vi "Attitude Indicator Facade.vi"(0 "Data In":T6, 2 "Display State In":T2={"Draw Options"={"Text Color"=16777238, "Wing Color"=16751616, "Dial Outline Color"=13816530, "Sky Color"=3381759, "Ground Color"=8213043, "Horizon Line Color"=16777225, "Outline Color"=0, "Dial Background Color"=5987163, "Draw Wings"=TRUE, "Draw Text"=TRUE, "Font Name"="Helvetica", "Angle units"=enum."Radians"}}, 3 "Container State":T5) -> (6 "Data Out":T6, 7 "Display State Out":T2={"Draw Options"={"Text Color"=16777238, "Wing Color"=16751616, "Dial Outline Color"=13816530, "Sky Color"=3381759, "Ground Color"=8213043, "Horizon Line Color"=16777225, "Outline Color"=0, "Dial Background Color"=5987163, "Draw Wings"=TRUE, "Draw Text"=TRUE, "Font Name"="Helvetica", "Angle units"=enum."Radians"}}, 8 "Action":T1)   [LabVIEW 2017, in "Attitude Indicator.xctl"]
uses:
  <vilib>/robotics/Controls/Attitude Indicator/Attitude Indicator.xctl
  <vilib>/robotics/Controls/Attitude Indicator/_Attitude Indicator Support Files/Attitude Indicator Data.ctl
  <vilib>/_xctls/Container State.ctl
  <vilib>/robotics/Controls/Attitude Indicator/_Attitude Indicator Support Files/Attitude Indicator State.ctl
  <vilib>/robotics/Controls/Attitude Indicator/Attitude Picture/Draw Options.ctl
  <vilib>/robotics/Controls/Utilities/Angle Units.ctl
  <vilib>/_xctls/Action.ctl
  <vilib>/_xctls/XControlSupport.lvlib
  <vilib>/robotics/Controls/Utilities/NI_Robotics_Control Utilities.lvlib
  <vilib>/robotics/Controls/Attitude Indicator/Attitude Picture/NI_Robotics_Attitude Picture.lvlib
panel:
  out "2D Picture":picture
types:
  T1 = typedef "XControlSupport.lvlib/Action.ctl" = cluster{"Data Changed?":bool, "State Changed?":bool, "Action Name":string}
  T2 = typedef "Attitude Indicator.xctl/Attitude Indicator State.ctl" = cluster{"Draw Options":T3}
  T3 = typedef "NI_Robotics_Attitude Picture.lvlib/Draw Options.ctl" = cluster{"Text Color":u32, "Wing Color":u32, "Dial Outline Color":u32, "Sky Color":u32, "Ground Color":u32, "Horizon Line Color":u32, "Outline Color":u32, "Dial Background Color":u32, "Draw Wings":bool, "Draw Text":bool, "Font Name":string, "Angle units":T4}
  T4 = typedef "NI_Robotics_Control Utilities.lvlib/Angle Units.ctl" = enum16{"Radians", "Degrees"}
  T5 = typedef "XControlSupport.lvlib/Container State.ctl" = cluster{"Indicator?":bool, "Run Mode?":bool, " Refnum":refnum<vi>}
  T6 = typedef "Attitude Indicator.xctl/Attitude Indicator Data.ctl" = cluster{"Roll":dbl, "Pitch":dbl}
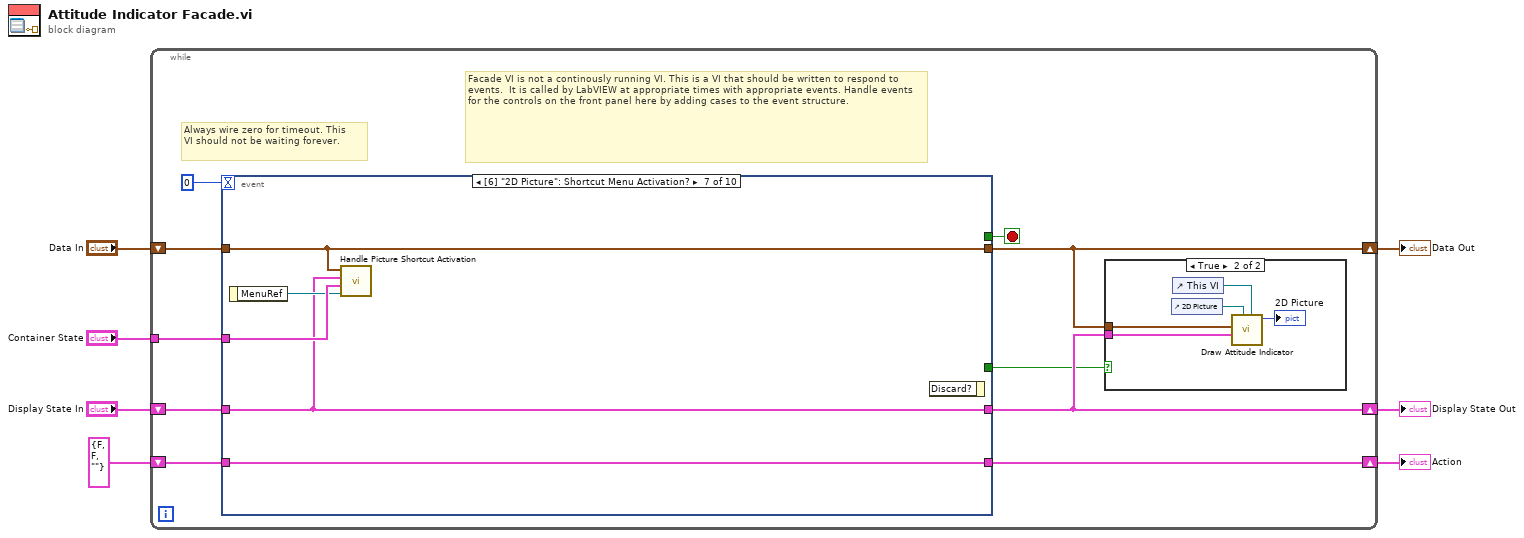
[diagram p0: block diagram]
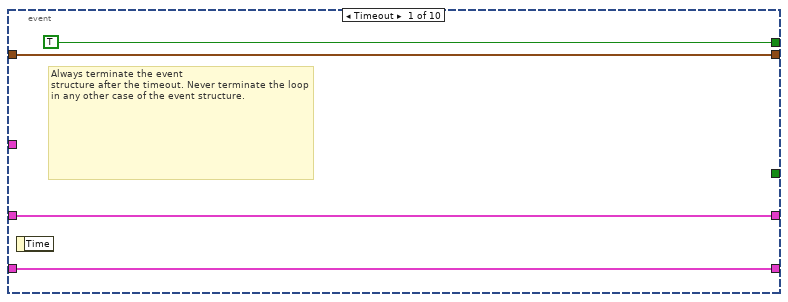
[diagram p3: hidden frame]
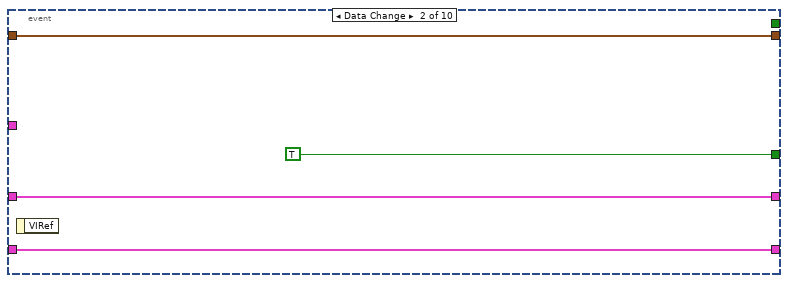
[diagram p4: hidden frame]
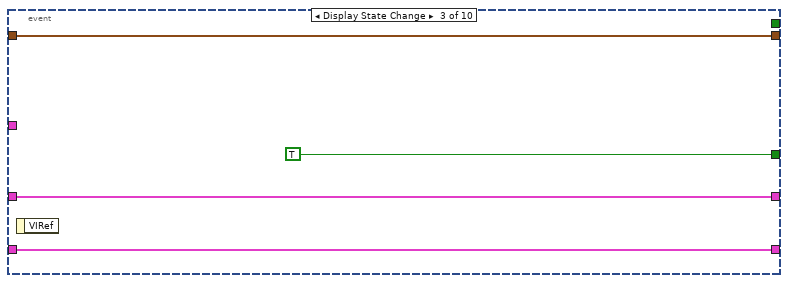
[diagram p5: hidden frame]
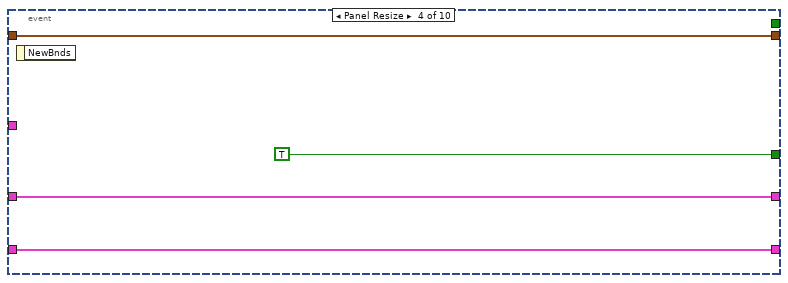
[diagram p6: hidden frame]
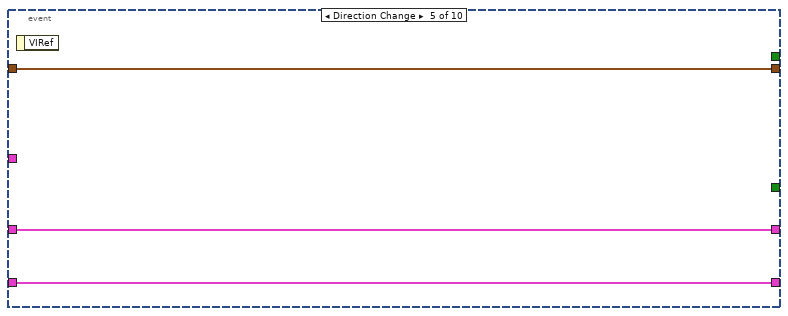
[diagram p7: hidden frame]
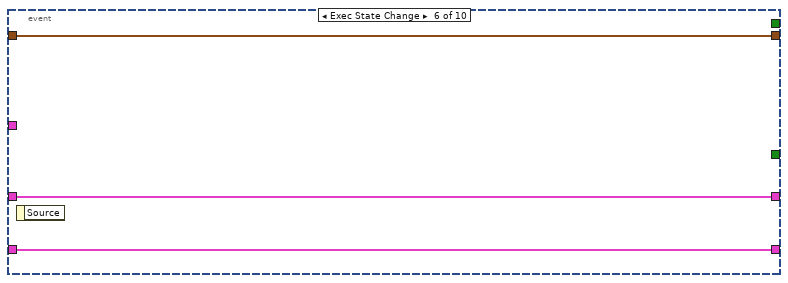
[diagram p8: hidden frame]
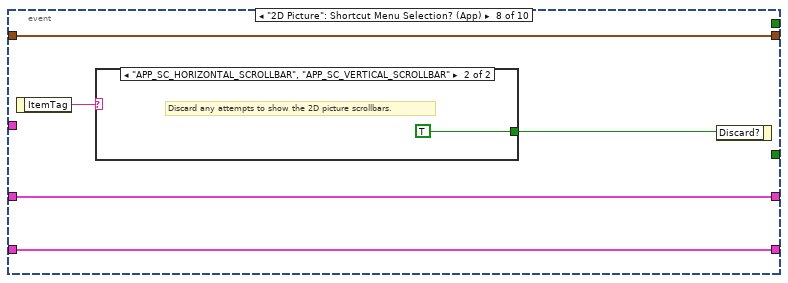
[diagram p9: hidden frame]
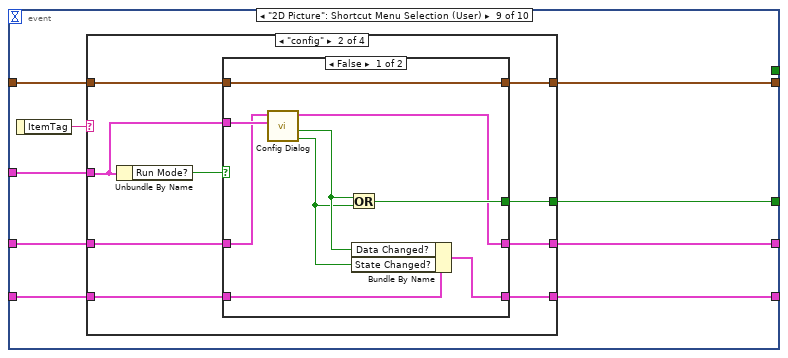
[diagram p11: hidden frame]
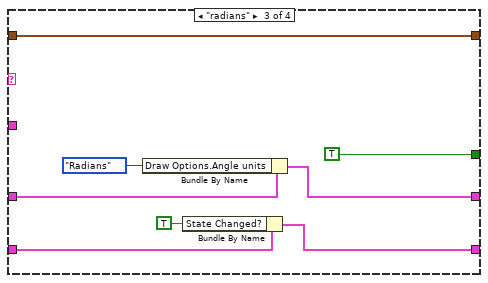
[diagram p14: hidden frame]
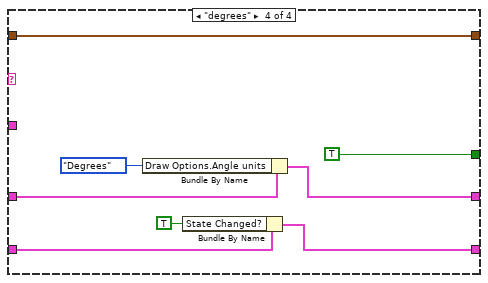
[diagram p15: hidden frame]
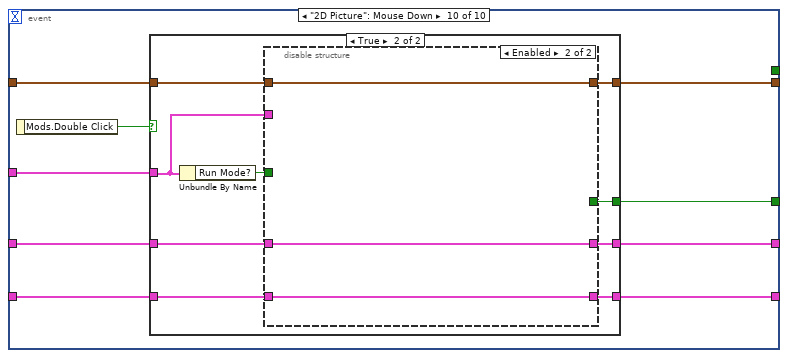
[diagram p16: hidden frame]
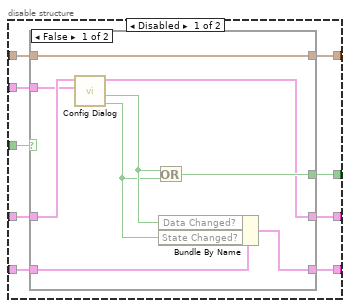
[diagram p18: hidden frame]
diagram:
  n1 = while {
    shift-right: [w10] -> w4
    shift-left: "Display State In" -> [w17]
    tunnel: "Container State" -> [w14]
    shift-right: [w11] -> w7
    shift-left: "Data In" -> [w13]
    shift-right: [w9] -> w1
    shift-left: T1 {"Data Changed?"=FALSE, "State Changed?"=FALSE, "Action Name"=""} ("Action") -> [w12]
    stop <- w16 stop-if-true
    # "Facade VI is not a continously running VI. This is a VI that should be written to respond to events.  It is called by LabVIEW at appropriate times with appropriate events. Handle events for the controls on the front panel here by adding cases to the event structure."
    # "Always wire zero for timeout. This\nVI should not be waiting forever."
    n2 = event shown="[6] \"2D Picture\": Shortcut Menu Activation?" {
      selector: _ -> [_ _ _ _ _ _ _ _ _ _]
      dyn-events: _ -> [_ _ _ _ _ _ _ _ _ _]
      timeout: 0 -> [_ _ _ _ _ _ _ _ _ _]
      tunnel: w17 -> [w25 w28 w32 w37 w41 w44 w45 w54 w61 w110]
      tunnel: [w25 w28 w32 w37 w41 w44 w45 w54 w60 w109] -> w10
      tunnel: [TRUE _ _ _ _ _ _ _ _ _] -> w16
      tunnel: w14 -> [_ _ _ _ _ _ w48 _ w56 w105]
      tunnel: w13 -> [w24 w29 w33 w38 w40 w43 w46 w53 w63 w112]
      tunnel: [w24 w29 w33 w38 w40 w43 w46 w53 w62 w111] -> w11
      tunnel: w12 -> [w23 w27 w31 w36 w39 w42 w49 w52 w59 w108]
      tunnel: [w23 w27 w31 w36 w39 w42 w49 w52 w58 w107] -> w9
      tunnel: [_ TRUE TRUE TRUE _ _ _ _ w57 w106] -> w8
      event Timeout {
        # "Always terminate the event\nstructure after the timeout. Never terminate the loop in any other case of the event structure."
        n3 = event-data() -> ()  [unwired: 1 in, 1 out]
      }
      event Data Change {
        n4 = event-data() -> ()  [unwired: 1 in, 1 out]
      }
      event Display State Change {
        n5 = event-data() -> ()  [unwired: 1 in, 1 out]
      }
      event Panel Resize {
        n6 = event-data() -> ()  [unwired: 1 in, 1 out]
      }
      event Direction Change {
        n7 = event-data() -> ()  [unwired: 1 in, 1 out]
      }
      event Exec State Change {
        n8 = event-data() -> ()  [unwired: 1 in, 1 out]
      }
      event "2D Picture": Shortcut Menu Activation? {
        n9 = event-data() -> ("MenuRef"=w47:refnum<k9>)  [unwired: 1 in]
        n10 = call <vilib>:"Handle Picture Shortcut Activation.vi"("MenuRef"=w47, "Container State"=w48, "state in"=w45, "data in"=w46) -> ()  [unwired: 8 in]
        n11 = event-data() -> ()  [unwired: 2 in, 1 out]
      }
      event "2D Picture": Shortcut Menu Selection? (App) {
        n12 = event-data() -> ("ItemTag"=w50:string)  [unwired: 1 in]
        n13 = case shown="\"APP_SC_HORIZONTAL_SCROLLBAR\", \"APP_SC_VERTICAL_SCROLLBAR\"" w50 {
          tunnel: [_ TRUE] -> w51
          frame Default {
          }
          frame "APP_SC_HORIZONTAL_SCROLLBAR", "APP_SC_VERTICAL_SCROLLBAR" {
            # "Discard any attempts to show the 2D picture scrollbars."
          }
        }
        n14 = event-data("Discard?"=w51) -> ()  [unwired: 1 in, 1 out]
      }
      event "2D Picture": Shortcut Menu Selection (User) {
        n15 = event-data() -> ("ItemTag"=w64:string)  [unwired: 1 in]
        n16 = case shown="\"config\"" w64 {
          tunnel: w63 -> [w67 w76 w96 w104]
          tunnel: [w67 w75 w96 w104] -> w62
          tunnel: w61 -> [w66 w74 w95 w103]
          tunnel: [w66 w73 w94 w102] -> w60
          tunnel: w59 -> [w65 w72 w92 w100]
          tunnel: [w65 w71 w91 w99] -> w58
          tunnel: [_ w70 TRUE TRUE] -> w57
          tunnel: w56 -> [_ w68 _ _]
          frame Default {
          }
          frame "config" {
            n17 = Unbundle By Name(w68) -> ("Run Mode?"=w69:bool)
            n18 = case shown="False" w69 {
              tunnel: w76 -> [w77 w88]
              tunnel: [w77 w88] -> w75
              tunnel: w74 -> [w78 w87]
              tunnel: [w80 w87] -> w73
              tunnel: w72 -> [w85 w86]
              tunnel: [w84 w86] -> w71
              tunnel: [w81 _] -> w70
              tunnel: w68 -> [w79 _]
              frame False {
                n19 = call <vilib>:"Config Dialog.vi"("Container State"=w79, "state in"=w78) -> ("state changed?"=w82:bool, "data changed?"=w83:bool, "state out"=w80:T2)  [unwired: 7 in]
                n20 = Or(x=w83, y=w82) -> (x .or. y?=w81:bool)
                n21 = Bundle By Name(cluster=w85, "Data Changed?"=w83, "State Changed?"=w82) -> (w84:T1)
              }
              frame True {
                # "Do not launch config dialog if xctl is in a running VI."
              }
            }
          }
          frame "radians" {
            n22 = Bundle By Name(cluster=w95, "Draw Options.Angle units"=Angle_Units."Radians") -> (w94:T2)
            n23 = Bundle By Name(cluster=w92, "State Changed?"=TRUE) -> (w91:T1)
          }
          frame "degrees" {
            n24 = Bundle By Name(cluster=w103, "Draw Options.Angle units"=Angle_Units."Degrees") -> (w102:T2)
            n25 = Bundle By Name(cluster=w100, "State Changed?"=TRUE) -> (w99:T1)
          }
        }
      }
      event "2D Picture": Mouse Down {
        n26 = event-data() -> ("Mods.Double Click"=w113:bool)  [unwired: 1 in]
        n27 = case shown="True" w113 {
          tunnel: w112 -> [w116 w125]
          tunnel: [w116 w124] -> w111
          tunnel: w110 -> [w115 w123]
          tunnel: [w115 w122] -> w109
          tunnel: w108 -> [w114 w121]
          tunnel: [w114 w120] -> w107
          tunnel: [_ w119] -> w106
          tunnel: w105 -> [_ w117]
          frame False {
          }
          frame True {
            n28 = Unbundle By Name(w117) -> ("Run Mode?"=w118:bool)
            n29 = disable-structure shown="Enabled" {
              disable-tunnel: w125 -> [w134 w149]
              disable-tunnel: [w133 w149] -> w124
              disable-tunnel: w123 -> [w132 w148]
              disable-tunnel: [w131 w148] -> w122
              disable-tunnel: w121 -> [w130 w147]
              disable-tunnel: [w129 w147] -> w120
              disable-tunnel: [w128 _] -> w119
              disable-tunnel: w118 -> [w127 _]
              disable-tunnel: w117 -> [w126 _]
              frame Disabled {
                n30 = case shown="False" w127 {
                  tunnel: w134 -> [w135 w146]
                  tunnel: [w135 w146] -> w133
                  tunnel: w132 -> [w137 w145]
                  tunnel: [w138 w145] -> w131
                  tunnel: w130 -> [w143 w144]
                  tunnel: [w142 w144] -> w129
                  tunnel: [w139 _] -> w128
                  tunnel: w126 -> [w136 _]
                  frame False {
                    n31 = call <vilib>:"Config Dialog.vi"("Container State"=w136, "state in"=w137) -> ("state changed?"=w140:bool, "data changed?"=w141:bool, "state out"=w138:T2)  [unwired: 7 in]
                    n32 = Or(x=w141, y=w140) -> (x .or. y?=w139:bool)
                    n33 = Bundle By Name(cluster=w143, "Data Changed?"=w141, "State Changed?"=w140) -> (w142:T1)
                  }
                  frame True {
                    # "Do not launch config dialog if xctl is in a running VI."
                  }
                }
              }
              frame Enabled {
              }
            }
          }
        }
      }
    }
    n34 = case shown="True" w8 {
      tunnel: w11 -> [_ w22]
      tunnel: w10 -> [_ w21]
      frame False {
      }
      frame True {
        n35 = control-ref of="2D Picture"() -> (w19:refnum<vi>)
        n36 = control-ref of="This VI"() -> (w18:refnum<vi>)
        n37 = call <vilib>:"Draw Attitude Indicator.vi"("FcdVI Refnum"=w18, "2D Picture"=w19, "State in"=w21, "Data in"=w22) -> ("Picture Out"=→"2D Picture":picture)  [unwired: 7 in]
      }
    }
  }
  "Display State Out" <- w4
  "Data Out" <- w7
  "Action" <- w1
